vi "Configure DC Current.vi"(0 "VISA resource name":refnum<visa-resource-name>, 1 "Enable Auto Range (T: Enable)":bool=TRUE, 3 "Auto-zero (1: On)":u16(ring)=1 format="%.0g" items=["Off", "On", "Once"], 4 "Manual Range (0 A)":dbl format="%#_6p", 5 "error in (no error)":errorcluster, 6 "Power Line Cycles (1.00)":dbl=1.0 format="%.2f", 7 "Sampling Interval (0.05)":dbl=0.05 min=0.0002 max=3600.0 step=0.0001 format="%.4f", 12 "Digits (5: 5 1/2)":u16(ring)=5 format="%.0g" items=["3 1/2 Digits"=3, "4 1/2 Digits"=4, "5 1/2 Digits"=5]) -> (14 "VISA resource name out":refnum<visa-resource-name>, 19 "error out":errorcluster)   [LabVIEW 2017, in "ADCMT7451_ADC.lvlib"]
doc: "Configures the measurement type, resolution, and range on the instrument."
uses:
  ADCMT7451_ADC.lvlib
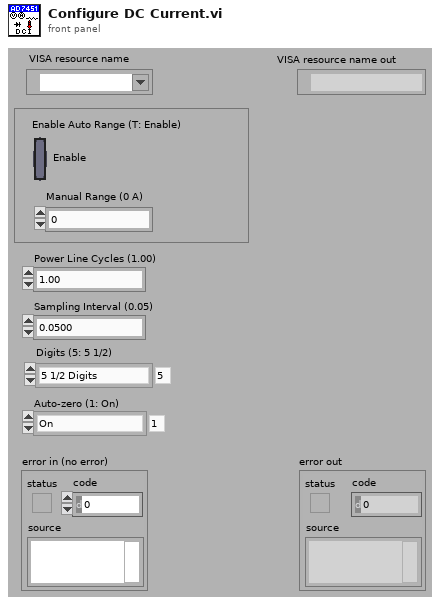
[diagram p1: front panel]
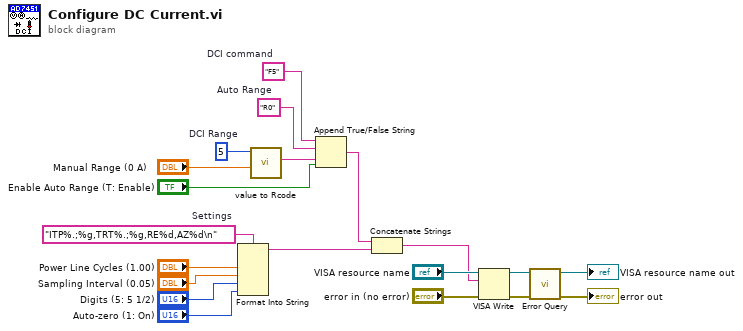
[diagram p0: block diagram]
diagram:
  w2 = "ITP%.;%g,TRT%.;%g,RE%d,AZ%d\n"  # Settings
  w8 = 5  # DCI Range
  w10 = "F5"  # DCI command
  w13 = "R0"  # Auto Range
  n1 = Format Into String(format string=w2, "Power Line Cycles (1.00)", "Sampling Interval (0.05)", "Digits (5: 5 1/2)", "Auto-zero (1: On)") -> (resulting string=w1:string)  [unwired: 2 in, 1 out]
  n2 = call "value to Rcode.vi"("Manual Range (0)"="Manual Range (0 A)", "Function (1: DC Volts)"=w8) -> ("Range Set Code"=w7:string)  [unwired: 9 in]
  n3 = Append True/False String(1:"Enable Auto Range (T: Enable)", 2:w7, 3:w13, 4:w10) -> (0:w12:string)
  n4 = Concatenate Strings(w12, w1) -> (w11:string)
  n5 = VISA Write(VISA resource name="VISA resource name", write buffer=w11, error in (no error)="error in (no error)") -> (VISA resource name out=w16:refnum<visa-resource-name>, error out=w15:errorcluster)  [unwired: 1 out]
  n6 = call "Error Query.vi"("error in (no error)"=w15, "VISA resource name"=w16) -> ("error out"=→"error out":errorcluster, "VISA resource name out"=→"VISA resource name out":refnum<visa-resource-name>)  [unwired: 6 in, 2 out]
